vi "事件结构（加法运算）.vi"() -> ()   [LabVIEW 2017]
panel:
  out "结果":dbl
  in  "b":dbl
  in  "a":dbl
  in  "停止":bool
  in  "加法运算开始":bool
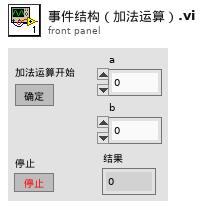
[diagram p1: front panel]
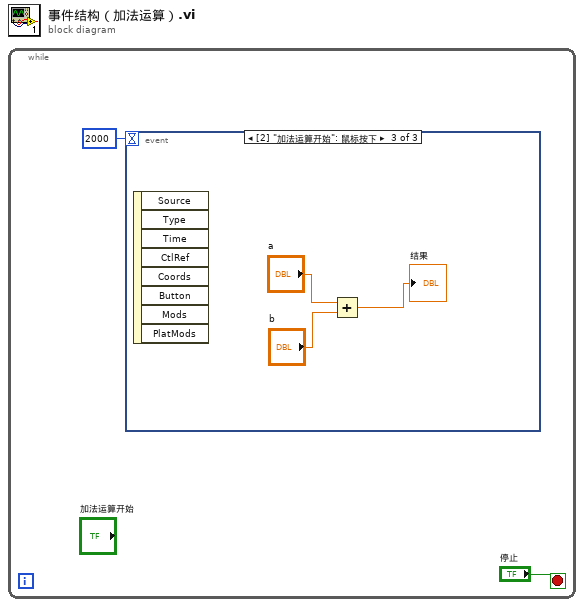
[diagram p0: block diagram]
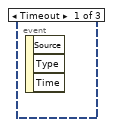
[diagram p2: hidden frame]
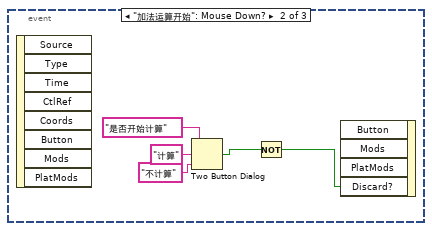
[diagram p3: hidden frame]
diagram:
  n1 = while {
    stop <- "停止" stop-if-true
    n2 = event shown="[2] \"加法运算开始\": 鼠标按下" {
      selector: _ -> [_ _ _]
      dyn-events: _ -> [_ _ _]
      timeout: 2000 -> [_ _ _]
      event Timeout {
        n3 = event-data() -> ()  [unwired: 1 in, 3 out]
      }
      event "加法运算开始": Mouse Down? {
        n4 = event-data() -> ()  [unwired: 1 in, 8 out]
        n5 = Two Button Dialog(message="是否开始计算" ("消息"), 1:"不计算" ("F按钮名称（“取消”）"), 2:"计算" ("T按钮名称（“确定”）")) -> (T button?=w7:bool)
        n6 = Not(x=w7) -> (.not. x?=w3:bool)
        n7 = event-data("Discard?"=w3) -> ()  [unwired: 4 in, 1 out]
      }
      event "加法运算开始": Mouse Down {
        n8 = event-data() -> ()  [unwired: 1 in, 8 out]
        n9 = Add(x="a", y="b") -> (x+y=→"结果":dbl)
      }
    }
  }
